vi "Clear Faults.vi"(8 "error in":errorcluster, 11 "Gantry in":refnum<class "Gantry.lvclass">) -> (0 "error out":errorcluster, 3 "Gantry out":refnum<class "Gantry.lvclass">)   [LabVIEW 2026, in "Gantry.lvclass"]
uses:
  Gantry.lvclass
  <instrlib>/Aerotech Automation1/Aerotech Automation1.lvlib
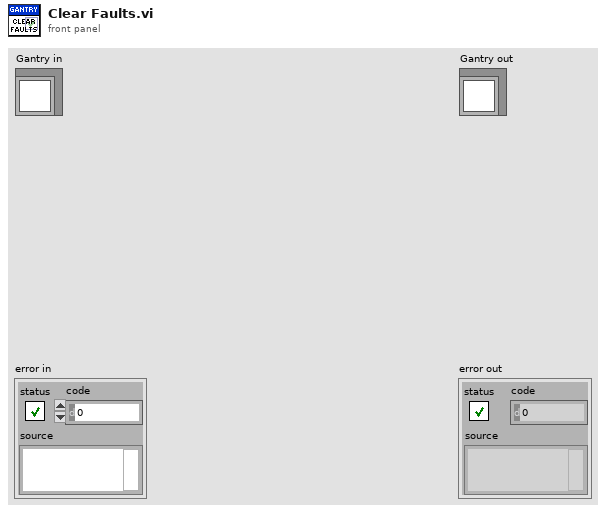
[diagram p1: front panel]
types:
  T1 = typedef "Virtual Modes.ctl" = enum16{"Nonvirtual", "Virtual"}
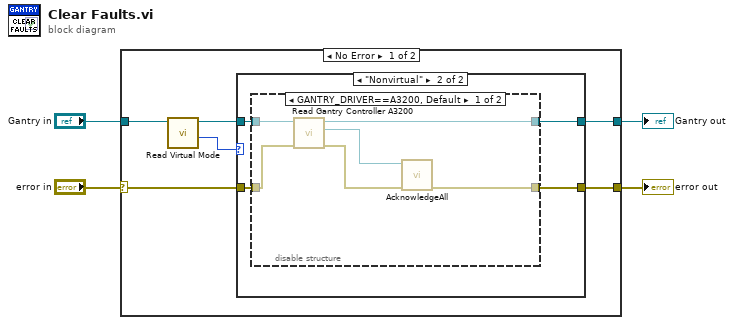
[diagram p0: block diagram]
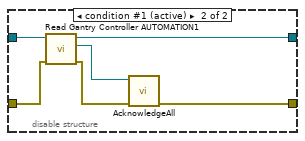
[diagram p3: hidden frame]
diagram:
  n1 = case shown="No Error" "error in" {
    selector: "error in" -> [w10 w30]
    tunnel: [w9 w30] -> w3
    tunnel: [w8 w29] -> w1
    tunnel: "Gantry in" -> [w7 w29]
    frame No Error {
      n2 = call-dynamic "Read Virtual Mode.vi"("Gantry in"=w7) -> ("Virtual Mode"=w5:T1, "Gantry out"=w6:refnum<class "Gantry.lvclass">)  [unwired: 7 in, 2 out]
      n3 = case shown="\"Nonvirtual\"" w5 {
        tunnel: w10 -> [w11 w13]
        tunnel: [w11 w16] -> w9
        tunnel: w6 -> [w12 w15]
        tunnel: [w12 w14] -> w8
        frame "Virtual" {
        }
        frame "Nonvirtual" {
          n4 = disable-structure shown="GANTRY_DRIVER==A3200, Default" {
            disable-tunnel: [w22 w24] -> w16
            disable-tunnel: w15 -> [w21 w26]
            disable-tunnel: [w20 w23] -> w14
            disable-tunnel: w13 -> [w19 w25]
            frame condition #0 {
              n5 = call "Read Gantry Controller A3200.vi"("error in (no error)"=w19, "Gantry in"=w21) -> ("error out"=w18:errorcluster, "A3200 controller out"=w17:refnum<k24>, "Gantry out"=w20:refnum<class "Gantry.lvclass">)  [unwired: 7 in]
              n6 = call <instrlib>:"AcknowledgeAll.vi"("error in (no error)"=w18, "controller in"=w17) -> ("error out"=w22:errorcluster)  [unwired: 8 in, 1 out]
            }
            frame condition #1 (active) {
              n7 = call "Read Gantry Controller AUTOMATION1.vi"("error in (no error)"=w25, "Gantry in"=w26) -> ("error out"=w27:errorcluster, "Controller AUTOMATION1"=w28:refnum<k24>, "Gantry out"=w23:refnum<class "Gantry.lvclass">)  [unwired: 7 in]
              n8 = call <instrlib>:"AcknowledgeAll.vi"("error in (no error)"=w27, "Controller Refnum"=w28) -> ("error out"=w24:errorcluster)  [unwired: 8 in, 1 out]
            }
          }
        }
      }
    }
    frame Error {
    }
  }
  "error out" <- w3
  "Gantry out" <- w1
